vi "Event Handler.vi"(0 "uService Template in":refnum<class "Simple Device Manager.lvclass">, 5 "Event type":T1=enum."Message", 7 "Item Name":string, 9 "Data":variant, 11 "error in (no error)":errorcluster) -> (4 "uService Template out":refnum<class "Simple Device Manager.lvclass">, 15 "error out":errorcluster)   [LabVIEW 2020, in "Simple Device Manager.lvlib" / "Simple Device Manager.lvclass"]
doc: "This VI is the event handler of the uService: every time an event is triggered to the uService, this VI is called.\nNote: here you can access the Actor/Class data, but it will be the one coming out from Init. You cannot modify the values.\nThree different events are supported:\nI) Button Pressed: get called on a GUI button pressed. Item Name is the name (label) of the button, Data is empty.\nII) Shared Variable Updated: get called when a SV you subscribed to is updated. Item Name is the name of the SV, and Data is the value (note: you need to convert it to the proper type).\nIII) Message: get called every time a user event is generated using Send Message to Event Handler. The values of Item Name and Data are the one given to the Send Message to Event Handler.\nIV) Ready to launch?: this frame get called every time a new Run is initiated. Each uService is responsible of performing a self check before giving back the green light for the Run to start."
uses:
  Simple Device Manager.lvclass
  TALOS/TALOS_PPL.lvlibp/Father of all uServices/Father of all uServices/Event Handler Items.ctl
  Consumer Case Selector.ctl
  TALOS/TALOS_PPL.lvlibp/Father of all uServices/Father of all uServices/Father of all uServices.lvclass
  TALOS/TALOS_PPL.lvlibp
  C:/LabVIEW Code/aegis-labview-code/TALOS/TALOS_PPL.lvlibp/Father of all uServices/Father of all uServices/Father of all uServices.lvclass
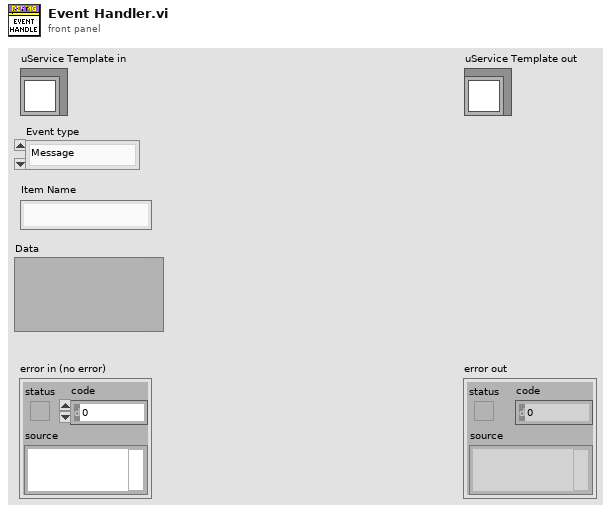
[diagram p1: front panel]
types:
  T1 = typedef "TALOS_PPL.lvlibp/Father of all uServices.lvlib/Father of all uServices.lvclass/Event Handler Items.ctl" = enum16{"Button Pressed", "Shared Variable Updated", "Message", "Ready to launch?", "Safe Mode", "Start RUN", "Stop RUN"}
  T2 = typedef "Simple Device Manager.lvlib/Simple Device Manager.lvclass/Consumer Case Selector.ctl" = enum16{"Set current", "Check status", "Check temperature"}
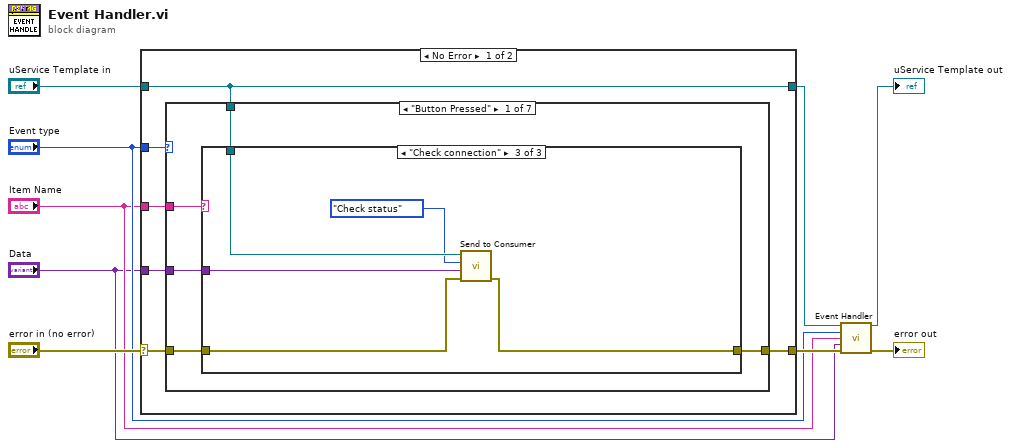
[diagram p0: block diagram]
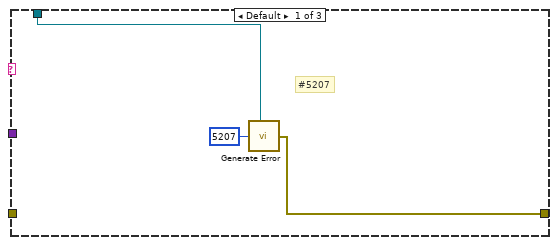
[diagram p2: hidden frame]
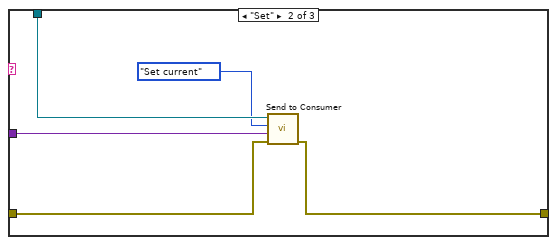
[diagram p3: hidden frame]
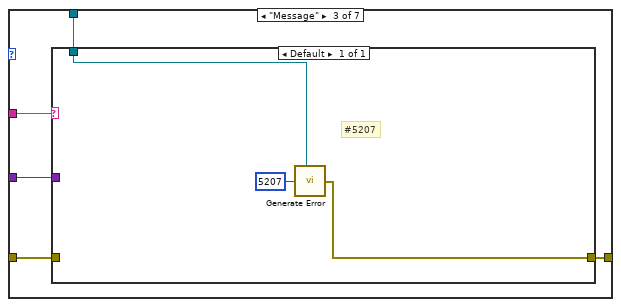
[diagram p5: hidden frame]
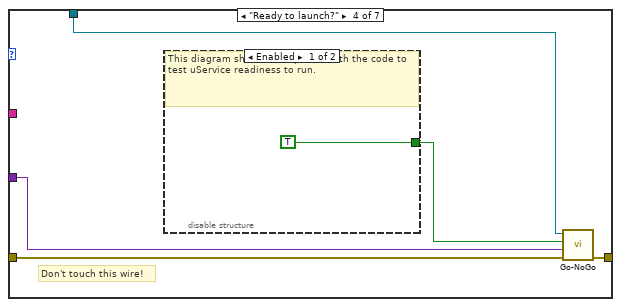
[diagram p6: hidden frame]
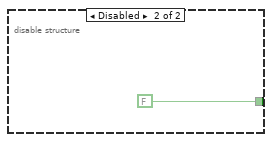
[diagram p7: hidden frame]
diagram:
  n1 = case shown="No Error" "error in (no error)" {
    selector: "error in (no error)" -> [w13 w54]
    tunnel: [w14 w54] -> w7
    tunnel: [w12 w53] -> w4
    tunnel: "uService Template in" -> [w12 w53]
    tunnel: "Event type" -> [w15 _]
    tunnel: "Item Name" -> [w11 _]
    tunnel: "Data" -> [w10 _]
    frame No Error {
      n2 = case shown="\"Button Pressed\"" w15 {
        tunnel: [w20 w34 w35 w46 w50 w51 w52] -> w14
        tunnel: w13 -> [w17 w34 w39 w47 w50 w51 w52]
        tunnel: w11 -> [w18 _ w38 _ _ _ _]
        tunnel: w12 -> [w19 _ w36 w45 _ _ _]
        tunnel: w10 -> [w16 _ w37 w43 _ _ _]
        frame "Button Pressed" {
          n3 = case shown="\"Check connection\"" w18 {
            tunnel: w17 -> [_ w27 w32]
            tunnel: [w21 w26 w31] -> w20
            tunnel: w19 -> [w22 w28 w33]
            tunnel: w16 -> [_ w25 w30]
            frame Default {
              # "#5207"
              n4 = call "Generate Error.vi"("Class"=w22, "Error Code"=5207) -> ("error out"=w21:errorcluster)  [unwired: 5 in]
            }
            frame "Set" {
              n5 = call "Send to Consumer.vi"("error in (no error)"=w27, "Data"=w25, "Case ID"=Consumer_Case_Selector."Set current" ("Consumer Case Selector"), "uService Template in"=w28) -> ("error out"=w26:errorcluster)  [unwired: 6 in, 1 out]
            }
            frame "Check connection" {
              n6 = call "Send to Consumer.vi"("error in (no error)"=w32, "Data"=w30, "Case ID"=Consumer_Case_Selector."Check status" ("Consumer Case Selector"), "uService Template in"=w33) -> ("error out"=w31:errorcluster)  [unwired: 6 in, 1 out]
            }
          }
        }
        frame "Shared Variable Updated" {
        }
        frame "Message" {
          n7 = case shown="Default" w38 {
            tunnel: w39 -> [_]
            tunnel: w37 -> [_]
            tunnel: w36 -> [w41]
            tunnel: [w40] -> w35
            frame Default {
              # "#5207"
              n8 = call "Generate Error.vi"("Class"=w41, "Error Code"=5207) -> ("error out"=w40:errorcluster)  [unwired: 5 in]
            }
          }
        }
        frame "Ready to launch?" {
          # "Don't touch this wire!"
          n9 = disable-structure shown="Enabled" {
            disable-tunnel: [TRUE ("Go?") FALSE ("Go?")] -> w44
            frame Enabled {
              # "This diagram should be replaced with the code to test uService readiness to run."
            }
            frame Disabled {
            }
          }
          n10 = call-dynamic "Go-NoGo.vi"("error in (no error)"=w47, "Go-NoGo Data"=w43, "Go?"=w44, "Father of all uServices in"=w45) -> ("error out"=w46:errorcluster)  [unwired: 6 in, 1 out]
        }
        frame "Safe Mode" {
          # "This case gets triggered"
        }
        frame "Start RUN" {
        }
        frame "Stop RUN" {
        }
      }
    }
    frame Error {
    }
  }
  n11 = call-parent "Event Handler.vi"("uService Template in"=w4, "Event type"="Event type", "Item Name"="Item Name", "Data"="Data", "error in (no error)"=w7) -> ("uService Template out"=→"uService Template out":refnum<class "Simple Device Manager.lvclass">, "error out"=→"error out":errorcluster)  [unwired: 9 in]
